vi "SetSourceAutorange.vi"(7 "SMU":T2, 8 "Error In":errorcluster, 9 "Enable?":bool, 10 "Source Function":T1, 11 "Keithley 2602 In":refnum<visa-resource-name>) -> (0 "Error Out":errorcluster, 3 "Keithley 2602 Out":refnum<visa-resource-name>)   [LabVIEW 2013, in "Keithley-2602.lvlib"]
uses:
  Keithley-2602.lvlib
  Controls/SMU.ctl
  Controls/SourceFunction.ctl
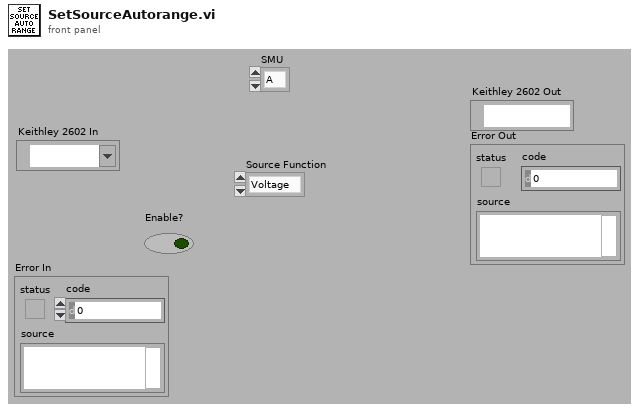
[diagram p1: front panel]
types:
  T1 = typedef "Keithley-2602.lvlib/SourceFunction.ctl" = enum16{"Voltage", "Current"}
  T2 = typedef "Keithley-2602.lvlib/SMU.ctl" = enum16{"A", "B"}
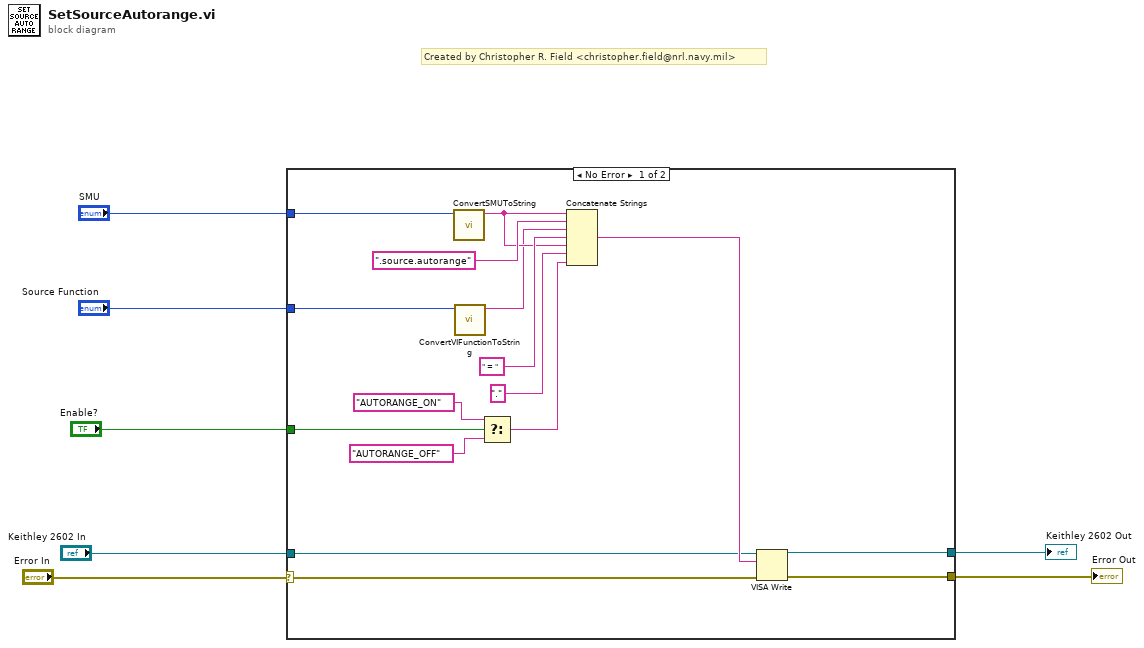
[diagram p0: block diagram]
diagram:
  # "Created by Christopher R. Field <christopher.field@nrl.navy.mil>"
  n1 = case shown="No Error" "Error In" {
    selector: "Error In" -> [w8 w24]
    tunnel: "Enable?" -> [w23 _]
    tunnel: "Keithley 2602 In" -> [w18 w25]
    tunnel: [w17 w25] -> w5
    tunnel: [w16 w24] -> w4
    tunnel: "SMU" -> [w10 _]
    tunnel: "Source Function" -> [w9 _]
    frame No Error {
      n2 = call "ConvertSMUToString.vi"("SMU"=w10) -> ("Channel"=w14:string)  [unwired: 10 in]
      n3 = call "ConvertVIFunctionToString.vi"("Function"=w9) -> ("Function (v or i)"=w11:string)  [unwired: 10 in]
      n4 = Select(t="AUTORANGE_ON", s=w23, f="AUTORANGE_OFF") -> (s? t:f=w12:string)
      n5 = Concatenate Strings(w14, ".source.autorange", w11, " = ", w14, "." ("string"), w12) -> (w19:string)
      n6 = VISA Write(VISA resource name=w18, write buffer=w19, error in (no error)=w8) -> (VISA resource name out=w17:refnum<visa-resource-name>, error out=w16:errorcluster)  [unwired: 1 out]
    }
    frame Error {
    }
  }
  "Keithley 2602 Out" <- w5
  "Error Out" <- w4
